vi "serial.vi"() -> ()   [LabVIEW 2020]
panel:
  out "vaia":dbl
  out "Waveform Chart":dbl(graph)
  out "vari":dbl
  out "var":dbl
  in  "Write":string
  in  "Enviar":bool
  out "Display":string
  in  "Close":bool
  in  "Open":bool
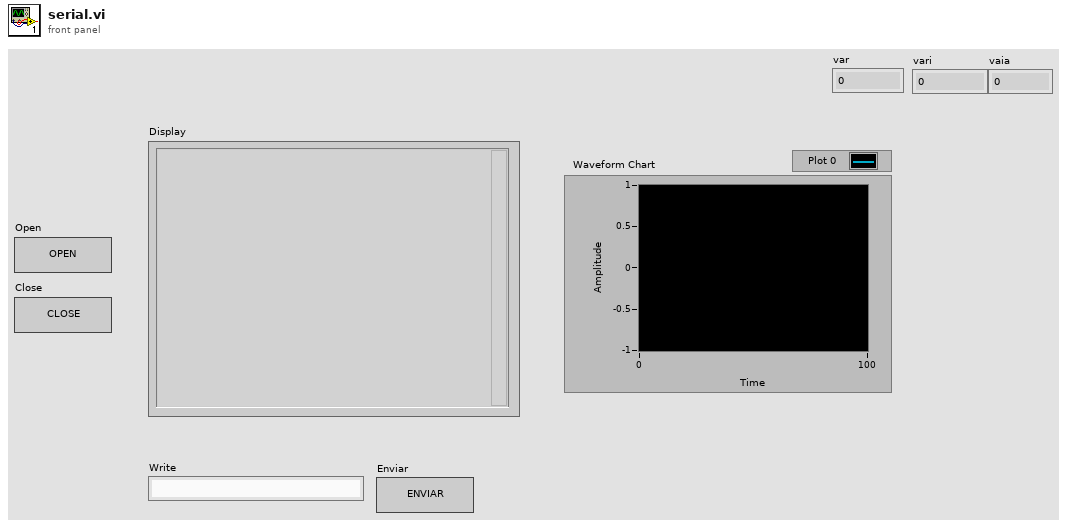
[diagram p1: front panel]
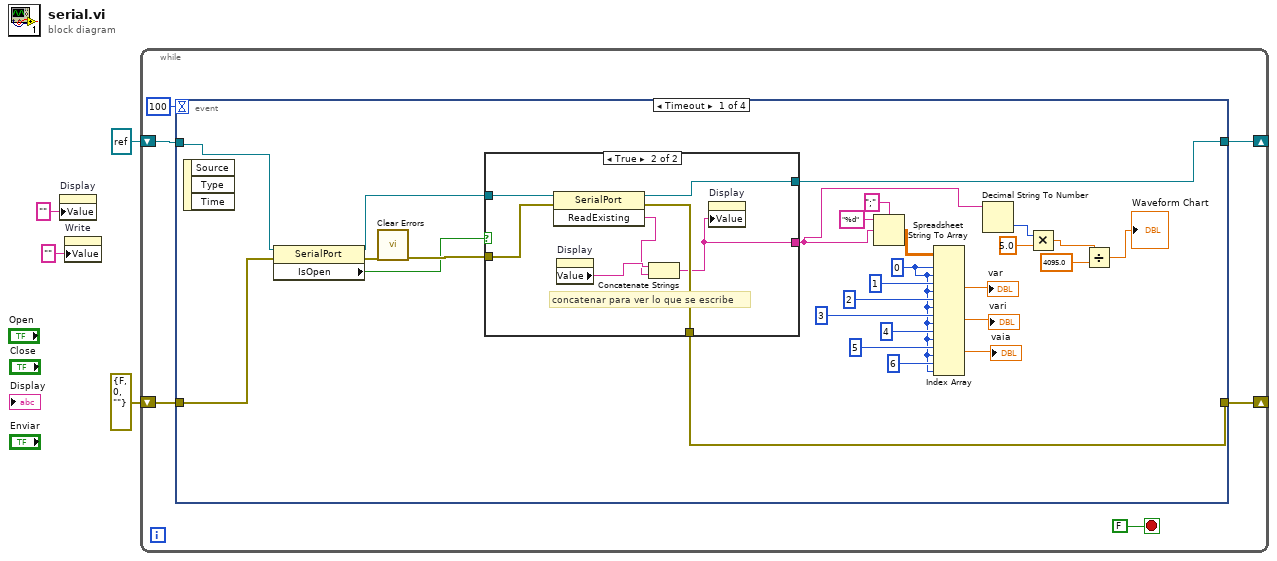
[diagram p0: block diagram]
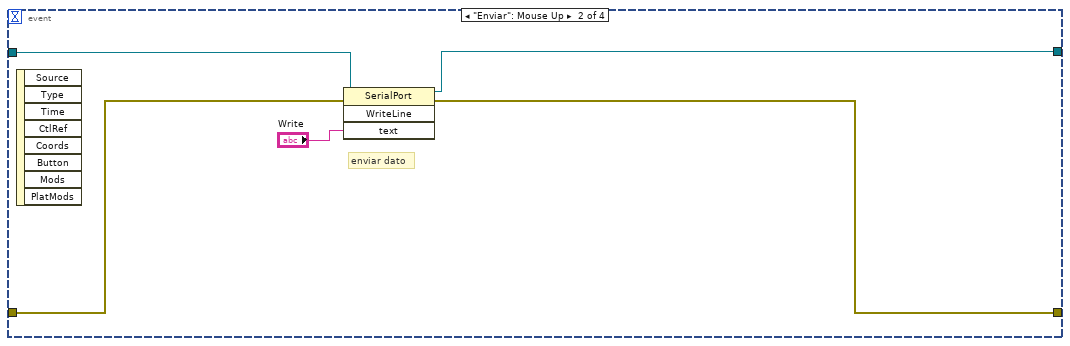
[diagram p3: hidden frame]
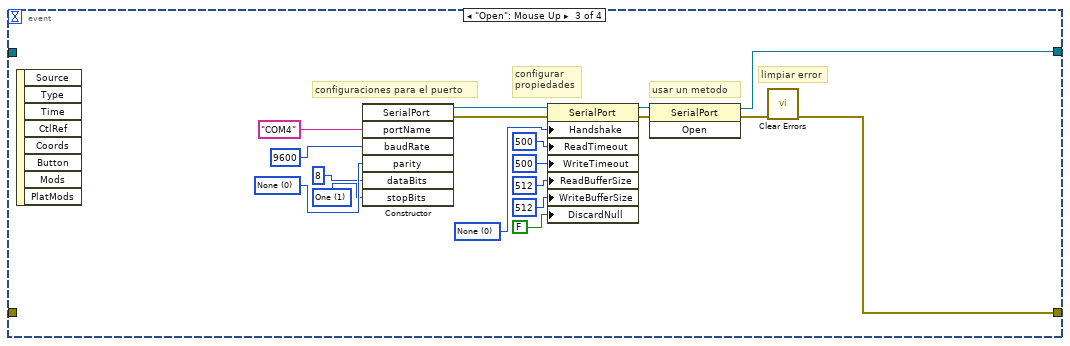
[diagram p4: hidden frame]
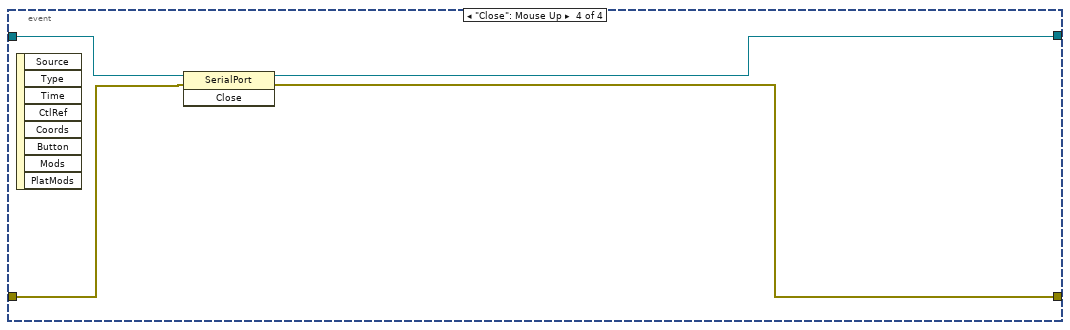
[diagram p5: hidden frame]
diagram:
  n1 = property on="Display" class="Str"("Value"="" ("Display")) -> ()  [unwired: 2 in, 2 out]
  n2 = property on="Write" class="Str"("Value"="" ("Write")) -> ()  [unwired: 2 in, 2 out]
  n3 = while {
    shift-right: [w9] -> _
    shift-left: refnum<k24> refnum ("new reference") -> [w7]
    shift-right: [w8] -> _
    shift-left: errorcluster {"status"=FALSE, "code"=0, "source"=""} ("error out") -> [w6]
    stop <- FALSE stop-if-true
    n4 = event shown="[0] Timeout" {
      selector: _ -> [_ _ _ _]
      dyn-events: _ -> [_ _ _ _]
      timeout: 100 -> [_ _ _ _]
      tunnel: [w37 w49 w53 w71] -> w9
      tunnel: [w36 w48 w52 w70] -> w8
      tunnel: w7 -> [w35 w51 _ w73]
      tunnel: w6 -> [w34 w50 _ w72]
      event Timeout {
        w18 = 0 ("index (row)")
        n5 = event-data() -> ()  [unwired: 1 in, 3 out]
        n6 = property class="SerialPort"(reference=w35, error in=w34) -> (reference out=w31:refnum<k24>, error out=w33:errorcluster, "IsOpen"=w30:bool)
        n7 = call <vilib>:"Clear Errors.vi"("error in (no error)"=w33) -> ("error out"=w32:errorcluster)  [unwired: 5 in, 1 out]
        n8 = case shown="True" w30 {
          tunnel: [w39 w46] -> w37
          tunnel: [w38 w45] -> w36
          tunnel: w32 -> [w38 w44]
          tunnel: w31 -> [w39 w43]
          tunnel: [_ w40] -> w21
          frame False {
          }
          frame True {
            # "concatenar para ver lo que se escribe"
            n9 = invoke class="SerialPort" method="ReadExisting"(reference=w43, error in=w44) -> (reference out=w46:refnum<k24>, error out=w45:errorcluster, "ReadExisting"=w41:string)  [unwired: 1 in]
            n10 = property on="Display" class="Str"() -> ("Value"=w42:string)  [unwired: 2 in, 2 out]
            n11 = Concatenate Strings(w42, w41) -> (w40:string)
            n12 = property on="Display" class="Str"("Value"=w40) -> ()  [unwired: 2 in, 2 out]
          }
        }
        n13 = Spreadsheet String To Array(delimiter (Tab)=";", format string="%d", spreadsheet string=w21) -> (array=w16:dbl[][])  [unwired: 1 in]
        n14 = Index Array(array=w16, index (row) #1=w18, index (col) #1=w18, index (row) #2=1 ("index (row)"), index (col) #2=w18, index (row) #3=2 ("index (row)"), index (col) #3=w18, index (row) #4=3 ("index (row)"), index (col) #4=w18, index (row) #5=4 ("index (row)"), index (col) #5=w18, index (row) #6=5 ("index (row)"), index (col) #6=w18, index (row) #7=6 ("index (row)"), index (col) #7=w18) -> (element #2=→"var":dbl, element #4=→"vari":dbl, element #6=→"vaia":dbl)  [unwired: 4 out]
        n15 = Decimal String To Number(string=w21) -> (number=w14:i32)  [unwired: 2 in, 1 out]
        n16 = Multiply(x=w14, y=5.0) -> (x*y=w12:dbl)
        n17 = Divide(x=w12, y=4095.0) -> (x/y=→"Waveform Chart":dbl)
      }
      event "Enviar": Mouse Up {
        # "enviar dato"
        n18 = event-data() -> ()  [unwired: 1 in, 8 out]
        n19 = invoke class="SerialPort" method="WriteLine"(reference=w51, error in=w50, "text"="Write") -> (reference out=w49:refnum<k24>, error out=w48:errorcluster)  [unwired: 1 in, 2 out]
      }
      event "Open": Mouse Up {
        w64 = 0 items=["None", "XOnXOff", "RequestToSend", "RequestToSendXOnXOff"] ("Handshake")
        w54 = 1 items=["None", "One", "Two", "OnePointFive"] ("stopBits")
        w56 = 0 items=["None", "Odd", "Even", "Mark", "Space"] ("parity")
        # "limpiar error"
        # "usar un metodo"
        # "configurar \npropiedades"
        # "configuraciones para el puerto"
        n20 = event-data() -> ()  [unwired: 1 in, 8 out]
        n21 = constructor class="SerialPort"("portName"="COM4", "baudRate"=9600, "parity"=w56, "dataBits"=8, "stopBits"=w54) -> (reference out=w65:refnum<k24>, error out=w66:errorcluster)  [unwired: 3 in, 6 out]
        n22 = property class="SerialPort"(reference=w65, error in=w66, "Handshake"=w64, "ReadTimeout"=500, "WriteTimeout"=500, "ReadBufferSize"=512, "WriteBufferSize"=512, "DiscardNull"=FALSE) -> (reference out=w67:refnum<k24>, error out=w68:errorcluster)
        n23 = invoke class="SerialPort" method="Open"(reference=w67, error in=w68) -> (reference out=w53:refnum<k24>, error out=w69:errorcluster)  [unwired: 1 in, 1 out]
        n24 = call <vilib>:"Clear Errors.vi"("error in (no error)"=w69) -> ("error out"=w52:errorcluster)  [unwired: 5 in, 1 out]
      }
      event "Close": Mouse Up {
        n25 = event-data() -> ()  [unwired: 1 in, 8 out]
        n26 = invoke class="SerialPort" method="Close"(reference=w73, error in=w72) -> (reference out=w71:refnum<k24>, error out=w70:errorcluster)  [unwired: 1 in, 1 out]
      }
    }
  }
